vi "Initialize.vi"(8 "error in (no error)":errorcluster, 10 "Transform":string, 11 "Transform in":refnum<class "Transform.lvclass">) -> (0 "error out":errorcluster, 3 "Transform out":refnum<class "Transform.lvclass">)   [LabVIEW 2019, in "Transform.lvclass"]
uses:
  Transform.lvclass
  <vilib>/Utility/error.llb/whitespace.ctl
  Transform.lvclass/Transform.ctl
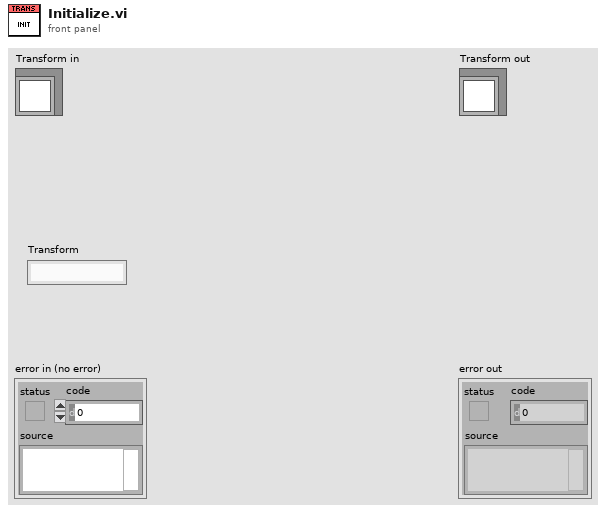
[diagram p1: front panel]
types:
  T1 = typedef "whitespace.ctl" = u16
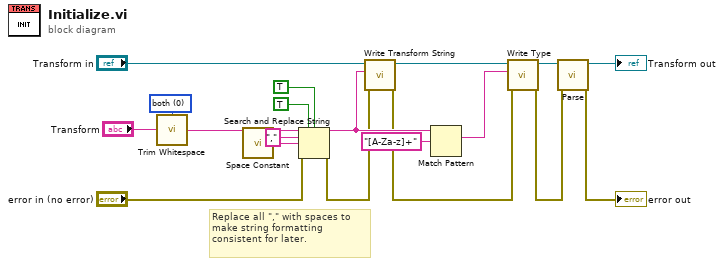
[diagram p0: block diagram]
diagram:
  w17 = T1 0 items=["both", "start of string", "end of string"] ("location (both)")
  # "Replace all \",\" with spaces to make string formatting consistent for later."
  n1 = call <vilib>:"Trim Whitespace.vi"("string"="Transform", "location (both)"=w17) -> ("trimmed string"=w6:string)
  n2 = call <vilib>:"Space Constant.vi"() -> ("String"=w9:string)
  n3 = Search and Replace String(replace all?=TRUE ("replace all? (F)"), case sensitive?=TRUE ("ignore case? (F)"), input string=w6, search string=",", replace string=w9, error in="error in (no error)") -> (result string=w5:string, error out=w4:errorcluster)  [unwired: 2 in, 2 out]
  n4 = call "Write Transform String.vi"("error in (no error)"=w4, "Transform String"=w5, "Transform in"="Transform in") -> ("error out"=w2:errorcluster, "Transform out"=w15:refnum<class "Transform.lvclass">)  [unwired: 7 in]
  n5 = Match Pattern(string=w5, regular expression="[A-Za-z]+") -> (match substring=w14:string)  [unwired: 1 in, 3 out]
  n6 = call "Write Type.vi"("error in (no error)"=w2, "Type"=w14, "Transform in"=w15) -> ("error out"=w11:errorcluster, "Transform out"=w13:refnum<class "Transform.lvclass">)  [unwired: 7 in]
  n7 = call-dynamic "Parse.vi"("error in (no error)"=w11, "Transform in"=w13) -> ("error out"=→"error out":errorcluster, "Transform out"=→"Transform out":refnum<class "Transform.lvclass">)  [unwired: 8 in]
